vi "Convert to Variable Cluster.vi"   [LabVIEW 2009]
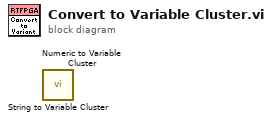
[diagram p0: block diagram]
diagram:
  n1 = call "String to Variable Cluster.vi"() -> ()  [unwired: 11 in, 1 out]
  n2 = call "Numeric to Variable Cluster.vi"() -> ()  [unwired: 11 in, 1 out]
